vi "Get Component Settings By Name.vi"(8 "error in (no error)":errorcluster, 10 "component name":string, 11 "Runtime Configuration in":refnum<class "Runtime Configuration.lvclass">) -> (0 "error out":errorcluster, 2 "component settings":T1, 3 "Runtime Configuration out":refnum<class "Runtime Configuration.lvclass">)   [LabVIEW 2017, in "DSF Core.lvlib" / "Runtime Configuration.lvclass"]
uses:
  Runtime Configuration.lvclass
  Typedefs/DSF Settings Info.ctl
  Typedefs/DSF Version Info.ctl
  Runtime Configuration.lvclass/Runtime Configuration.ctl
  DSF Core.lvlib
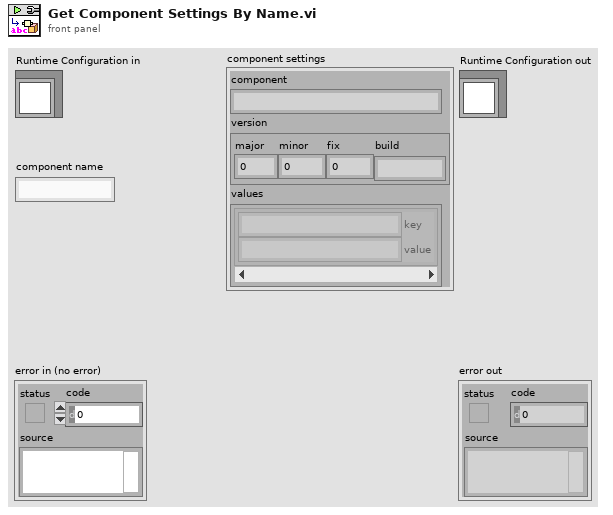
[diagram p1: front panel]
types:
  T1 = typedef "DSF Core.lvlib/DSF Settings Info.ctl" = cluster{"component":string, "version":T2, "values":cluster{"key":string, "value":string}[]}
  T2 = typedef "DSF Core.lvlib/DSF Version Info.ctl" = cluster{"major":u32, "minor":u32, "fix":u32, "build":string}
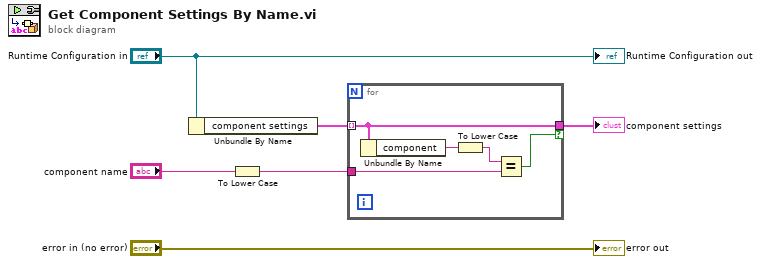
[diagram p0: block diagram]
diagram:
  n1 = Unbundle By Name("Runtime Configuration in") -> ("component settings"=w4:T1[])
  n2 = To Lower Case(string="component name") -> (all lower case string=w2:string)
  n3 = for {
    tunnel: w4 -> [w11] mode=indexing
    tunnel: w2 -> [w8]
    tunnel: [w11] -> w1 if=w7
    n4 = Unbundle By Name(w11) -> ("component"=w10:string)
    n5 = To Lower Case(string=w10) -> (all lower case string=w9:string)
    n6 = Equal?(x=w9, y=w8) -> (x = y?=w7:bool)
  }
  "component settings" <- w1
  "error out" <- "error in (no error)"
  "Runtime Configuration out" <- "Runtime Configuration in"
